vi "Read Status.vi"(8 "error in (no error)":errorcluster, 11 "Sample Line in":refnum<class "Sample Line.lvclass">) -> (0 "error out":errorcluster, 2 "Status":T1, 3 "Sample Line out":refnum<class "Sample Line.lvclass">)   [LabVIEW 2015, in "cRIO-Carbondioxide.lvlib" / "CO2-Actor.lvlib" / "Sample Line.lvclass"]
uses:
  Sample Line.lvclass
  Controls/Sample Line State Enumerator.ctl
  Sample Line.lvclass/Sample Line.ctl
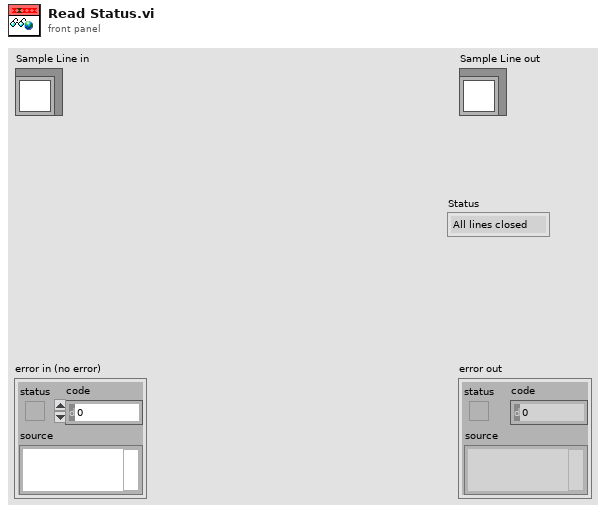
[diagram p1: front panel]
types:
  T1 = typedef "Sample Line State Enumerator.ctl" = enum16{"All lines closed", "Sample line 1.", "Sample line 2.", "Sample line 3.", "Sample line 4.", "Sample line 5.", "Out of range"}
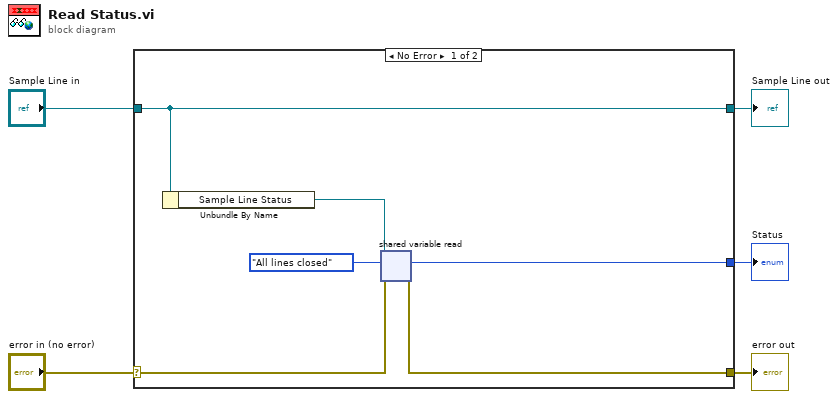
[diagram p0: block diagram]
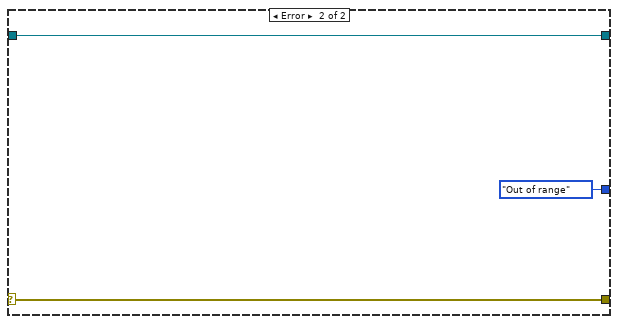
[diagram p2: hidden frame]
diagram:
  n1 = case shown="No Error" "error in (no error)" {
    selector: "error in (no error)" -> [w9 w14]
    tunnel: [w8 w14] -> w4
    tunnel: [w11 w13] -> w2
    tunnel: "Sample Line in" -> [w11 w13]
    tunnel: [w6 Sample_Line_State_Enumerator."Out of range" ("Enum")] -> w1
    frame No Error {
      n2 = Unbundle By Name(w11) -> ("Sample Line Status"=w10:refnum<k21>)
      n3 = shared-variable-read(w10, w9, Sample_Line_State_Enumerator."All lines closed" ("Enum")) -> (w8:errorcluster, w6:T1)  [unwired: 2 out]
    }
    frame Error {
    }
  }
  "error out" <- w4
  "Sample Line out" <- w2
  "Status" <- w1
